vi "子vi-路径-初始数据.vi"(11 "密码文件(789.whd)":string="789.whd") -> (1 "密码文件路径":path, 2 "用户名密码":cluster{"操作人员":string[][], "管理人员":string[][]}, 3 "T文件不存在":bool, 7 "原始路径":path)   [LabVIEW 2018]
panel:
  out "错误输出":errorcluster
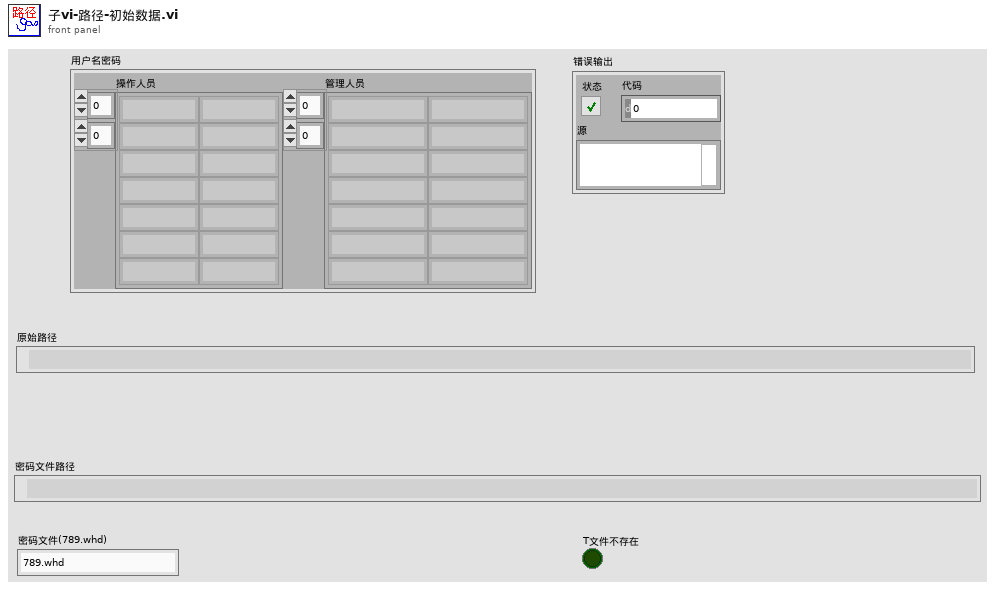
[diagram p1: front panel]
types:
  T1 = enum32{"invalid app kind", "Development System", "Run Time System", "Student Edition", "Embedded LabVIEW", "Evaluation", "Custom"}
  T2 = enum16{"open", "replace", "create", "open or create", "replace or create", "replace or create with confirmation"}
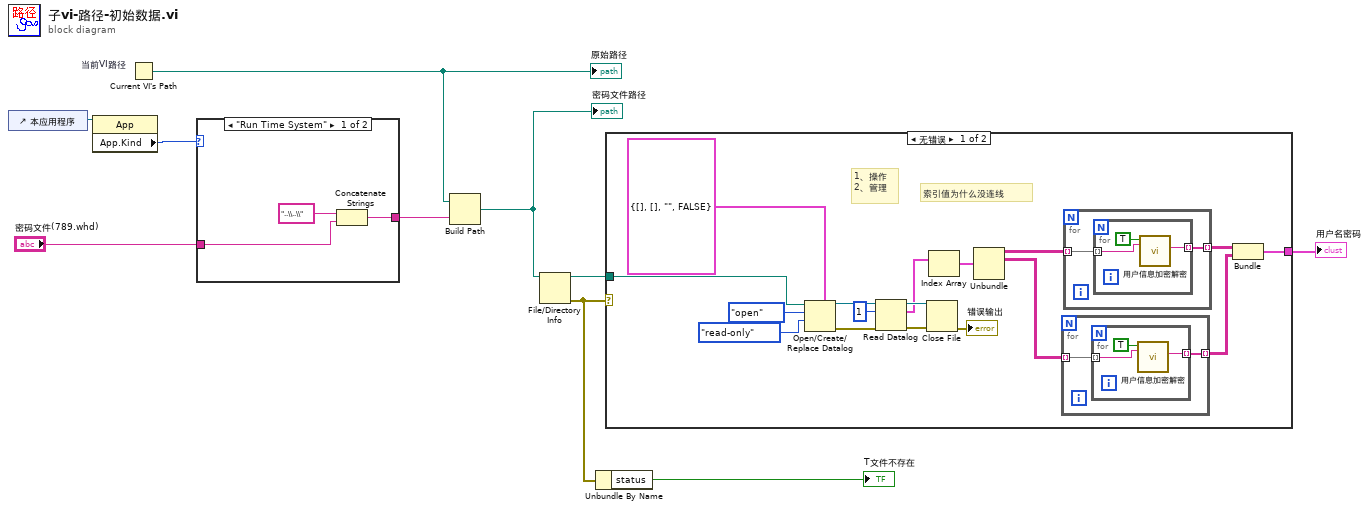
[diagram p0: block diagram]
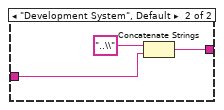
[diagram p3: hidden frame]
diagram:
  n1 = control-ref of="本应用程序"() -> (w10:refnum<vi>)
  n2 = property class="App"(reference=w10) -> ("App.Kind"=w9:T1)  [unwired: 1 in, 2 out]
  n3 = Current VI's Path "当前VI路径"() -> (path=w8:path)
  "原始路径" <- w8
  n4 = case shown="\"Run Time System\"" w9 {
    tunnel: [w12 w15] -> w7
    tunnel: "密码文件(789.whd)" -> [w11 w14]
    frame "Run Time System" {
      n5 = Concatenate Strings("..\\..\\" ("名称或相对路径"), w11) -> (w12:string)
    }
    frame "Development System", Default {
      n6 = Concatenate Strings("..\\" ("名称或相对路径"), w14) -> (w15:string)
    }
  }
  n7 = Build Path(base path=w8, name or relative path=w7) -> (appended path=w4:path)
  "密码文件路径" <- w4
  n8 = File/Directory Info(path=w4) -> (path out=w5:path, error out=w3:errorcluster)  [unwired: 1 in, 5 out]
  n9 = Unbundle By Name(w3) -> ("status"=→"T文件不存在":bool)
  n10 = case shown="无错误" w3 {
    tunnel: w5 -> [w25 _]
    tunnel: [w18 _] -> w1
    frame No Error {
      # "索引值为什么没连线"
      # "1、操作\n2、管理"
      n11 = Open/Create/Replace Datalog(5:cluster{string[][], string[][], string, bool} {[], [], "", FALSE}, 9:enum16{"read/write", "read-only", "write-only"}."read-only" ("权限(0:read/write)"), 10:T2."open" ("操作(0:open)"), 11:w25) -> (0:w31:errorcluster, 3:w29:refnum<k1>)  [unwired: 2 in, 1 out]
      n12 = Read Datalog(4:w31, 6:1 ("总数(1)"), 7:w29) -> (0:w33:errorcluster, 2:w24:cluster{string[][], string[][], string, bool}[], 3:w32:refnum<k1>)
      n13 = Close File(refnum=w32, error in=w33) -> (error out=→"错误输出":errorcluster)  [unwired: 1 out]
      n14 = Index Array(array=w24) -> (element=w21:cluster{string[][], string[][], string, bool})  [unwired: 1 in]
      n15 = Unbundle(w21) -> (w23:string[][], w22:string[][])  [unwired: 2 out]
      n16 = for {
        tunnel: w22 -> [w35] mode=indexing
        tunnel: [w34] -> w19 mode=indexing
        n17 = for {
          tunnel: w35 -> [w37] mode=indexing
          tunnel: [w36] -> w34 mode=indexing
          n18 = call "用户信息加密解密.vi"("加密字符串_in"=w37, "T解密-F加密"=TRUE) -> ("原始字符串_out"=w36:string)  [unwired: 4 in, 1 out]
        }
      }
      n19 = for {
        tunnel: w23 -> [w40] mode=indexing
        tunnel: [w39] -> w20 mode=indexing
        n20 = for {
          tunnel: w40 -> [w42] mode=indexing
          tunnel: [w41] -> w39 mode=indexing
          n21 = call "用户信息加密解密.vi"("加密字符串_in"=w42, "T解密-F加密"=TRUE) -> ("原始字符串_out"=w41:string)  [unwired: 4 in, 1 out]
        }
      }
      n22 = Bundle(w20, w19) -> (w18:cluster{string[][], string[][]})  [unwired: 1 in]
    }
    frame Error {
    }
  }
  "用户名密码" <- w1
